vi "Генератор 2D массива.vi"(0 "Y range":cluster{"X max":dbl, "X min":dbl, "X max":dbl}={"X max"=40.0, "X min"=-40.0, "X max"=40.0} {"X max" format="%.2f"; "X max" format="%.2f"; "X min" format="%.2f"}, 1 "Y resolution":i32=100, 2 "wave definitions":T2(array[cluster])=[{"X Freq"=1.0, "Initial X"=-20.0, "Y Freq"=2.0, "Initial Y"=20.0, "Magnitude"=1.0}, {"X Freq"=2.0, "Initial X"=20.0, "Y Freq"=0.5, "Initial Y"=-10.0, "Magnitude"=1.0}] {"Magnitude" format="%.2f"; "Initial Y" format="%.2f"; "Y Freq" format="%.2f"; "Initial X" format="%.2f"; "X Freq" format="%.2f"}, 3 "X range":cluster{"X max":dbl, "X min":dbl, "X min":dbl}={"X max"=40.0, "X min"=-40.0, "X min"=-40.0} {"X min" format="%.2f"; "X max" format="%.2f"; "X min" format="%.2f"}, 4 "X resolution":i32=100) -> (5 "scaling factors":T1={"Xo/deltaX"={"Xo"=40.0, "deltaX"=-40.0}, "Yo/deltaY"={"Yo"=40.0, "deltaY"=-40.0}, "Z range"={"minimum"=40.0, "maximum"=-40.0, "increment"=-40.0}} {"Z range"."increment" format="%.2f"; "Z range"."minimum" format="%.2f"; "Z range"."maximum" format="%.2f"; "Yo/deltaY"."Yo" format="%.2f"; "Yo/deltaY"."deltaY" format="%.2f"; "Xo/deltaX"."Xo" format="%.2f"; "Xo/deltaX"."deltaX" format="%.2f"}, 6 "data":dbl[][](graph))   [LabVIEW 2017]
doc: "This VI is a subVI to an exercise in the LabVIEW Basics I course.\n\nThis VI is called by Intensity Graph Example.vi. It uses an intensity graph to display a simulated wave interference pattern."
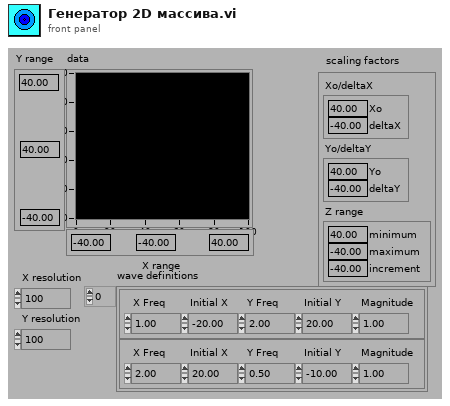
[diagram p1: front panel]
types:
  T1 = cluster{"Xo/deltaX":cluster{"Xo":dbl, "deltaX":dbl}, "Yo/deltaY":cluster{"Yo":dbl, "deltaY":dbl}, "Z range":cluster{"minimum":dbl, "maximum":dbl, "increment":dbl}}
  T2 = cluster{"X Freq":dbl, "Initial X":dbl, "Y Freq":dbl, "Initial Y":dbl, "Magnitude":dbl}[]
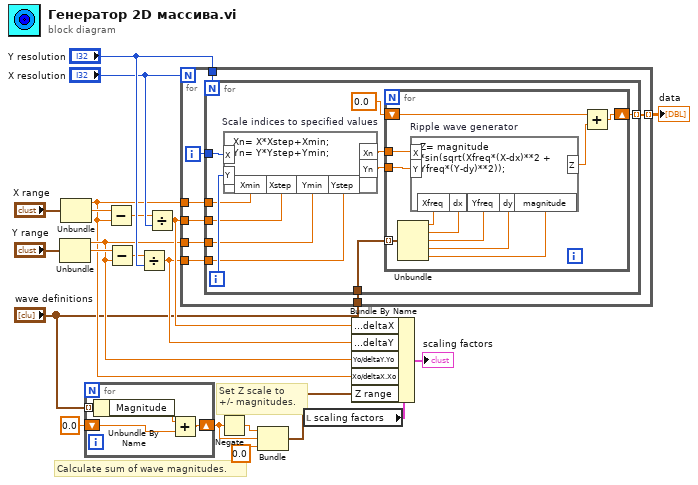
[diagram p0: block diagram]
diagram:
  # "Set Z scale to \n+/- magnitudes."
  # "Calculate sum of wave magnitudes."
  n1 = Unbundle("Y range") -> ("X max"=w10:dbl, "X min"=w14:dbl)  [unwired: 1 out]
  n2 = Unbundle("X range") -> ("X max"=w9:dbl, "X min"=w15:dbl)  [unwired: 1 out]
  n3 = for {
    tunnel: "wave definitions" -> [w25] mode=indexing
    shift-right: [w24] -> w3
    shift-left: 0.0 -> [w22]
    n4 = Unbundle By Name(w25) -> ("Magnitude"=w23:dbl)
    n5 = Add(x=w23, y=w22) -> (x+y=w24:dbl)
  }
  n6 = Subtract(x=w15, y=w9) -> (x-y=w13:dbl)
  n7 = Subtract(x=w14, y=w10) -> (x-y=w18:dbl)
  n8 = Divide(x=w18, y="Y resolution") -> (x/y=w11:dbl)
  n9 = Divide(x=w13, y="X resolution") -> (x/y=w12:dbl)
  n10 = for {
    N: "X resolution" -> [_]
    tunnel: "Y resolution" -> [w32]
    tunnel: [w31] -> w19 mode=indexing
    tunnel: w9 -> [w30]
    tunnel: w10 -> [w29]
    tunnel: w12 -> [w28]
    tunnel: w11 -> [w27]
    tunnel: "wave definitions" -> [w26]
    i -> [w33]
    n11 = for {
      N: w32 -> [_]
      tunnel: w33 -> [w43]
      tunnel: [w42] -> w31 mode=indexing
      tunnel: w30 -> [w41]
      tunnel: w29 -> [w39]
      tunnel: w28 -> [w37]
      tunnel: w27 -> [w36]
      tunnel: w26 -> [w35]
      i -> [w44]
      n12 = formula code="Xn= X*Xstep+Xmin;\nYn= Y*Ystep+Ymin;" "Scale indices to specified values"("X"=w43, "Xstep"=w37, "Xmin"=w41, "Y"=w44, "Ystep"=w36, "Ymin"=w39) -> ("Xn"=w38:dbl, "Yn"=w40:dbl)
      n13 = for {
        shift-right: [w55] -> w42
        shift-left: 0.0 -> [w53]
        tunnel: w38 -> [w52]
        tunnel: w40 -> [w51]
        tunnel: w35 -> [w50] mode=indexing
        n14 = Unbundle(w50) -> ("X Freq"=w49:dbl, "Initial X"=w48:dbl, "Y Freq"=w47:dbl, "Initial Y"=w46:dbl, "Magnitude"=w45:dbl)
        n15 = formula code="Z= magnitude *sin(sqrt(Xfreq*(X-dx)**2 + Yfreq*(Y-dy)**2));" "Ripple wave generator"("X"=w52, "Y"=w51, "Xfreq"=w49, "dx"=w48, "Yfreq"=w47, "dy"=w46, "magnitude"=w45) -> ("Z"=w54:dbl)
        n16 = Add(x=w53, y=w54) -> (x+y=w55:dbl)
      }
    }
  }
  "data" <- w19
  n17 = Negate(x=w3) -> (-x=w4:dbl)
  n18 = Bundle(w4, w3, 0.0) -> (w1:cluster{dbl, dbl, dbl})  [unwired: 1 in]
  n19 = local read "scaling factors"() -> (w7:T1)
  n20 = Bundle By Name(cluster=w7, "Xo/deltaX.deltaX"=w12, "Yo/deltaY.deltaY"=w11, "Yo/deltaY.Yo"=w10, "Xo/deltaX.Xo"=w9, "Z range"=w1) -> (→"scaling factors":T1)
